vi "Draw Scalable Border.vi"(8 "error in (no error)":errorcluster, 9 "Bounds":cluster{"Width":u32, "Height":u32}, 10 "Position":cluster{"Left":i32, "Top":i32}, 11 "8 Points Border in":refnum<class "8 Points Border.lvclass">) -> (0 "error out":errorcluster, 2 "Border out":picture, 3 "8 Points Border out":refnum<class "8 Points Border.lvclass">)   [LabVIEW 2015, in "8 Points Border.lvclass"]
uses:
  8 Points Border.lvclass
panel:
  # "NOTICE -- YOU MUST LEAVE THIS NOTICE IN PLACE.\n\nCopyright (c) 2017, LIANG LIU Shawn.Liu.cn@gmail.com\nAll rights reserved.\n\nRedistribution and use in source and binary forms, with or without modification, are permitted provided that the following conditions are met:\n-Redistributions of source code must retain the above copyright notice, this list of conditions and the following disclaimer.\n-Redistributions in binary form must reproduce the above copyright notice, this list of conditions and the following disclaimer in the documentation and/or other materials provided with the distribution.\n-Neither the name of the eLp nor the names of its contributors may be used to endorse or promote products derived from this software without specific prior written permission.\n\nTHIS SOFTWARE IS PROVIDED BY THE COPYRIGHT HOLDERS AND CONTRIBUTORS \"AS IS\" AND ANY EXPRESS OR IMPLIED WARRANTIES, INCLUDING, BUT NOT LIMITED TO, THE IMPLIED WARRANTIES OF MERCHANTABILITY AND FITNESS FOR A PARTICULAR PURPOSE ARE DISCLAIMED. IN NO EVENT SHALL THE COPYRIGHT HOLDER OR CONTRIBUTORS BE LIABLE FOR ANY DIRECT, INDIRECT, INCIDENTAL, SPECIAL, EXEMPLARY, OR CONSEQUENTIAL DAMAGES (INCLUDING, BUT NOT LIMITED TO, PROCUREMENT OF SUBSTITUTE GOODS OR SERVICES; LOSS OF USE, DATA, OR PROFITS; OR BUSINESS INTERRUPTION) HOWEVER CAUSED AND ON ANY THEORY OF LIABILITY, WHETHER IN CONTRACT, STRICT LIABILITY, OR TORT (INCLUDING NEGLIGENCE OR OTHERWISE) ARISING IN ANY WAY OUT OF THE USE OF THIS SOFTWARE, EVEN IF ADVISED OF THE POSSIBILITY OF SUCH DAMAGE."
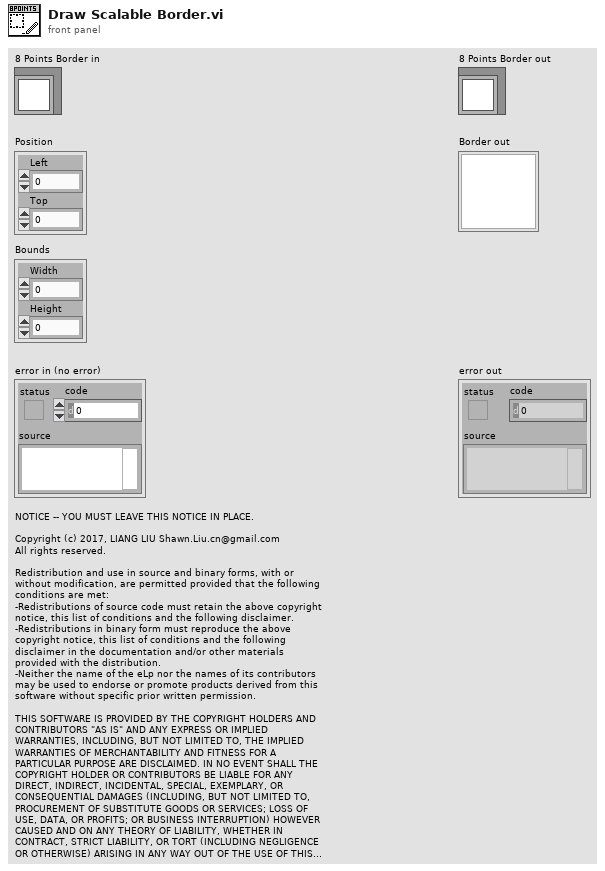
[diagram p1: front panel]
types:
  T1 = cluster{"left":i16, "top":i16, "right":i16, "bottom":i16}
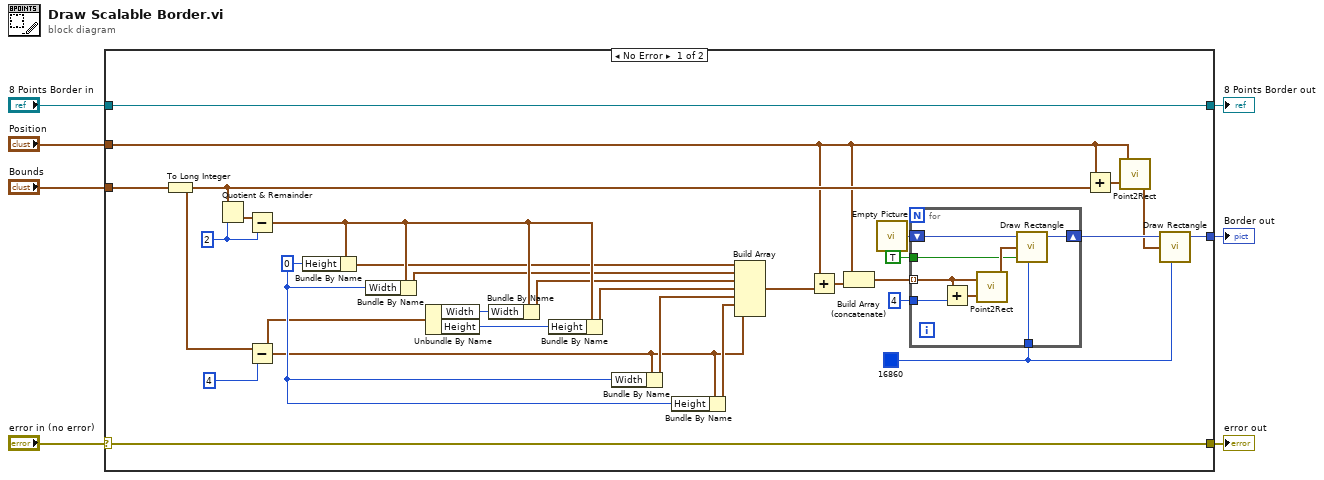
[diagram p0: block diagram]
diagram:
  n1 = case shown="No Error" "error in (no error)" {
    selector: "error in (no error)" -> [w37 w47]
    tunnel: "8 Points Border in" -> [w8 w46]
    tunnel: [w8 w46] -> w3
    tunnel: [w36 _] -> w2
    tunnel: [w37 w47] -> w1
    tunnel: "Bounds" -> [w10 _]
    tunnel: "Position" -> [w9 _]
    frame No Error {
      w16 = u32 16860
      w29 = 0 ("Width")
      w34 = 2
      n2 = To Long Integer(number=w10) -> (32bit integer=w14:cluster{"Width":i32, "Height":i32})
      n3 = Quotient & Remainder(x=w14, y=w34) -> (floor(x/y)=w35:cluster{"Width":i32, "Height":i32})  [unwired: 1 out]
      n4 = Subtract(x=w35, y=w34) -> (x-y=w31:cluster{"Width":i32, "Height":i32})
      n5 = Subtract(x=w14, y=4) -> (x-y=w22:cluster{"Width":i32, "Height":i32})
      n6 = Bundle By Name(cluster=w31, "Height"=w29) -> (w28:cluster{"Width":i32, "Height":i32})
      n7 = Bundle By Name(cluster=w31, "Width"=w29) -> (w25:cluster{"Width":i32, "Height":i32})
      n8 = Unbundle By Name(w22) -> ("Width"=w33:i32, "Height"=w32:i32)
      n9 = Bundle By Name(cluster=w31, "Width"=w33) -> (w24:cluster{"Width":i32, "Height":i32})
      n10 = Bundle By Name(cluster=w31, "Height"=w32) -> (w23:cluster{"Width":i32, "Height":i32})
      n11 = Bundle By Name(cluster=w22, "Width"=w29) -> (w27:cluster{"Width":i32, "Height":i32})
      n12 = Bundle By Name(cluster=w22, "Height"=w29) -> (w26:cluster{"Width":i32, "Height":i32})
      n13 = Build Array(w28, w25, w24, w23, w27, w26, w22) -> (w21:cluster{"Width":i32, "Height":i32}[])
      n14 = Add(x=w9, y=w21) -> (x+y=w20:cluster{i32, i32}[])
      n15 = Build Array (concatenate)(w9, w20) -> (w15:cluster{"Left":i32, "Top":i32}[])
      n16 = call "Empty Picture"() -> ("empty picture"=w13:picture)
      n17 = for {
        tunnel: w15 -> [w44] mode=indexing
        shift-right: [w41] -> w18
        shift-left: w13 -> [w45]
        tunnel: TRUE -> [w40]
        tunnel: w16 -> [w39]
        tunnel: 4 -> [w38]
        n18 = Add(x=w44, y=w38) -> (x+y=w43:cluster{"Left":i32, "Top":i32})
        n19 = call <vilib>:"Point2Rect.vi"("point b"=w43, "point a"=w44) -> ("rect"=w42:T1)
        n20 = call <vilib>:"Draw Rectangle.vi"("picture"=w45, "rect"=w42, "fill?(F)"=w40, "color(black)"=w39) -> ("new picture"=w41:picture)  [unwired: 5 in]
      }
      n21 = Add(x=w9, y=w14) -> (x+y=w17:cluster{i32, i32})
      n22 = call <vilib>:"Point2Rect.vi"("point b"=w17, "point a"=w9) -> ("rect"=w11:T1)
      n23 = call <vilib>:"Draw Rectangle.vi"("picture"=w18, "rect"=w11, "color(black)"=w16) -> ("new picture"=w36:picture)  [unwired: 6 in]
    }
    frame Error {
    }
  }
  "error out" <- w1
  "8 Points Border out" <- w3
  "Border out" <- w2
